vi "Wago Input Image.vi"(8 "Error In":errorcluster, 10 "Wago Data Input":T1 {"Input Process Image"."Software Constants"."Room PID Settings"."Room Dehumid Temperature I (*RM Dehum I1)" max=30000 step=1; "Input Process Image"."Software Constants"."Room PID Settings"."Room Dehumid Temperature P (*RM Dehum P1)" max=30000 step=1; "Input Process Image"."Software Constants"."Room PID Settings"."Room Cool Temperature I (*RM Cool I1)" max=30000 step=1; "Input Process Image"."Software Constants"."Room PID Settings"."Room Cool Temperature P (*RM Cool P1)" max=30000 step=1; "Input Process Image"."Software Constants"."Room PID Settings"."Room Heat I (*RM Heat I1)" max=30000 step=1; "Input Process Image"."Software Constants"."Room PID Settings"."Room Heat P (*RM Heat P1)" max=30000 step=1; "Input Process Image"."Software Constants"."Room PID Settings"."Room Humidity I (*RM Hum I1)" max=30000 step=1; "Input Process Image"."Software Constants"."Room PID Settings"."Room Humidity P (*RM Hum P1)" max=30000 step=1; "Input Process Image"."Software Constants"."Room PID Settings"."Room Dry I (*RM Dry I1)" max=30000 step=1; "Input Process Image"."Software Constants"."Room PID Settings"."Room Dry P(*RM Dry P1)" max=30000 step=1}, 11 "Modbus Master in":refnum<class "Modbus Master.lvclass">) -> (0 "Error Out":errorcluster, 2 "Wago Data Output":T1 {"Input Process Image"."Software Constants"."Room PID Settings"."Room Dehumid Temperature I (*RM Dehum I1)" max=30000 step=1; "Input Process Image"."Software Constants"."Room PID Settings"."Room Dehumid Temperature P (*RM Dehum P1)" max=30000 step=1; "Input Process Image"."Software Constants"."Room PID Settings"."Room Cool Temperature I (*RM Cool I1)" max=30000 step=1; "Input Process Image"."Software Constants"."Room PID Settings"."Room Cool Temperature P (*RM Cool P1)" max=30000 step=1; "Input Process Image"."Software Constants"."Room PID Settings"."Room Heat I (*RM Heat I1)" max=30000 step=1; "Input Process Image"."Software Constants"."Room PID Settings"."Room Heat P (*RM Heat P1)" max=30000 step=1; "Input Process Image"."Software Constants"."Room PID Settings"."Room Humidity I (*RM Hum I1)" max=30000 step=1; "Input Process Image"."Software Constants"."Room PID Settings"."Room Humidity P (*RM Hum P1)" max=30000 step=1; "Input Process Image"."Software Constants"."Room PID Settings"."Room Dry I (*RM Dry I1)" max=30000 step=1; "Input Process Image"."Software Constants"."Room PID Settings"."Room Dry P(*RM Dry P1)" max=30000 step=1}, 3 "Modbus master out":refnum<class "Modbus Master.lvclass">)   [LabVIEW 2016]
uses:
  <vilib>/NI/Modbus Library/API/Master/Modbus Master.lvclass
  Type Definitions/Wago Main Control.ctl
  Type Definitions/Wago Output Data Process Image.ctl
  Type Definitions/Wago Room Condtions.ctl
  Type Definitions/Wago Door Relays.ctl
  Type Definitions/Wago Contactor Settings.ctl
  Type Definitions/Wago Ground Leakage.ctl
  Type Definitions/Wago Input Process Image.ctl
  Type Definitions/Wago Room PID Settings.ctl
  Type Definitions/Wago Measured Input Data.ctl
  Type Definitions/Wago Room Setpoint Targets.ctl
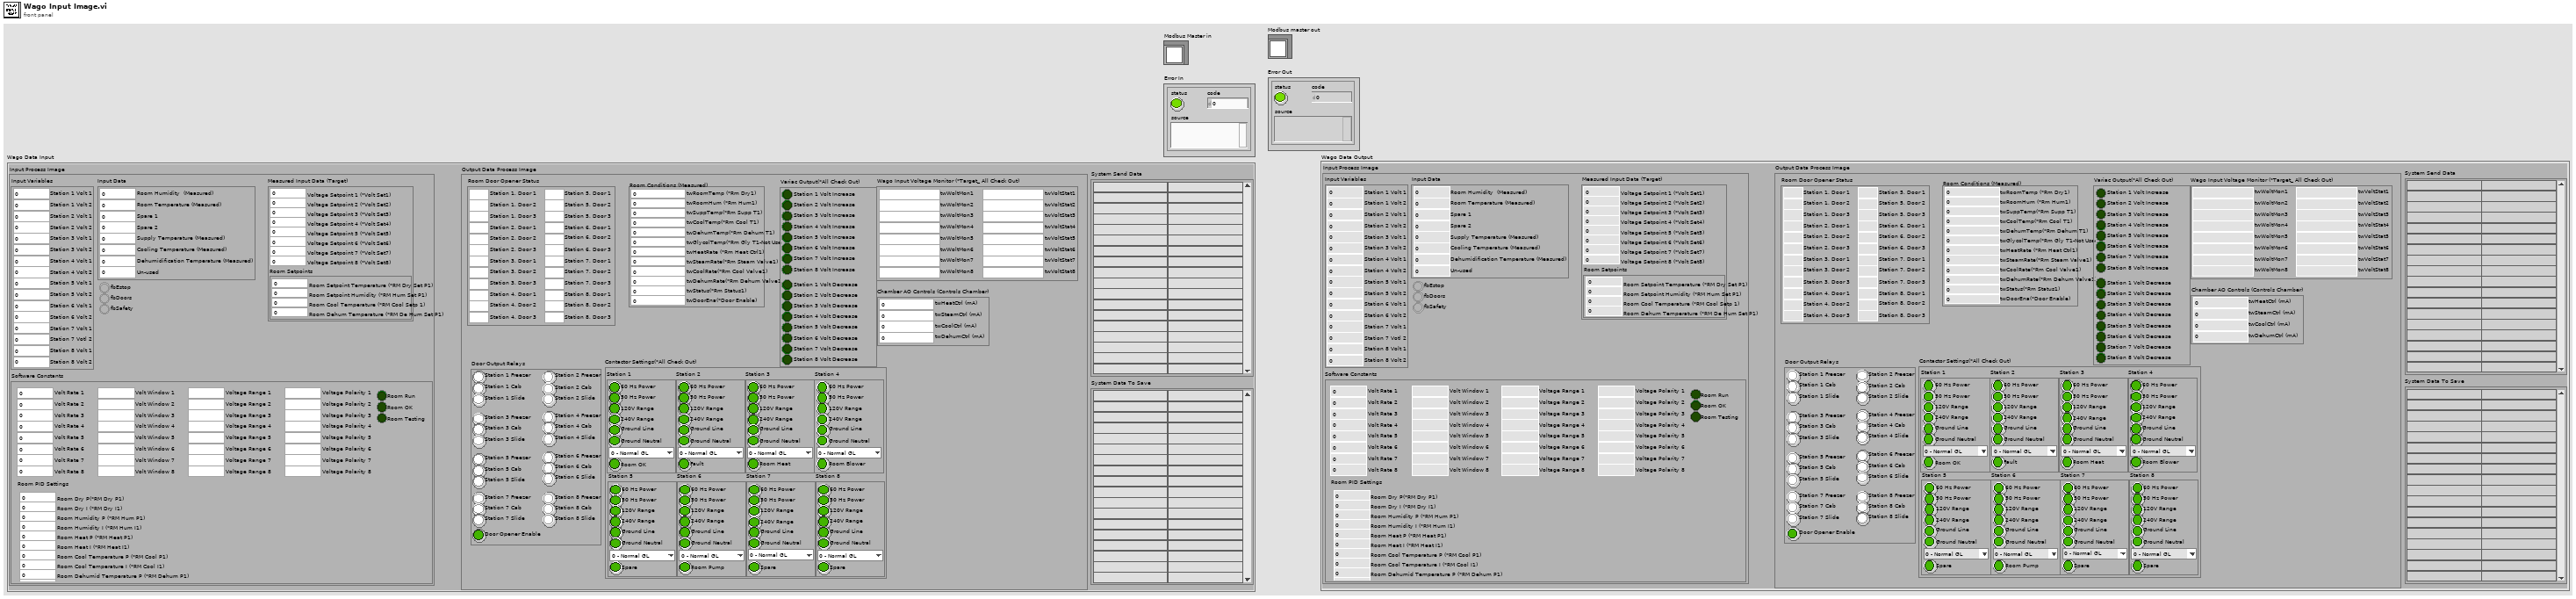
[diagram p1: front panel]
types:
  T1 = typedef "Wago Main Control.ctl" = cluster{"Output Data Process Image":T2, "Input Process Image":T7, "System Send Data":string[][], "System Data To Save":string[][]}
  T2 = typedef "Wago Output Data Process Image.ctl" = cluster{"Room Door Opener Status":cluster{"Station 1, Door 1":u16, "Station 1, Door 2":u16, "Station 1, Door 3":u16, "Station 2, Door 1":u16, "Station 2, Door 2":u16, "Station 2, Door 3":u16, "Station 3, Door 1":u16, "Station 3, Door 2":u16, "Station 3, Door 3":u16, "Station 4, Door 1":u16, "Station 4, Door 2":u16, "Station 4, Door 3":u16, "Station 5, Door 1":u16, "Station 5, Door 2":u16, "Station 5, Door 3":u16, "Station 6, Door 1":u16, "Station 6, Door 2":u16, "Station 6, Door 3":u16, "Station 7, Door 1":u16, "Station 7, Door 2":u16, "Station 7, Door 3":u16, "Station 8, Door 1":u16, "Station 8, Door 2":u16, "Station 8, Door 3":u16}, "Room Conditions (Measured)":T3, "Chamber AO Controls (Controls Chamber)":cluster{"twDehumCtrl (mA)":u16, "twCoolCtrl (mA)":u16, "twSteamCtrl (mA)":u16, "twHeatCtrl (mA)":u16}, "Variac Output(*All Check Out)":cluster{"Station 1 Volt Increase":bool, "Station 1 Volt Decrease":bool, "Station 2 Volt Increase":bool, "Station 2 Volt Decrease":bool, "Station 3 Volt Increase":bool, "Station 3 Volt Decrease":bool, "Station 4 Volt Increase":bool, "Station 4 Volt Decrease":bool, "Station 5 Volt Increase":bool, "Station 5 Volt Decrease":bool, "Station 6 Volt Increase":bool, "Station 6 Volt Decrease":bool, "Station 7 Volt Increase":bool, "Station 7 Volt Decrease":bool, "Station 8 Volt Increase":bool, "Station 8 Volt Decrease":bool}, "Door Output Relays":T4, "Wago Input Voltage Monitor (*Target_ All Check Out)":cluster{"twWoltMon1":dbl, "twWoltMon2":dbl, "twWoltMon3":dbl, "twWoltMon4":dbl, "twWoltMon5":dbl, "twWoltMon6":dbl, "twWoltMon7":dbl, "twWoltMon8":dbl, "twVoltStat1":u16, "twVoltStat2":u16, "twVoltStat3":u16, "twVoltStat4":u16, "twVoltStat5":u16, "twVoltStat6":u16, "twVoltStat7":u16, "twVoltStat8":u16}, "Contactor Settings(*All Check Out)":T5}
  T3 = typedef "Wago Room Condtions.ctl" = cluster{"twDoorEna(*Door Enable)":u16, "twStatus(*Rm Status1)":u16, "twRoomTemp (*Rm Dry1)":dbl, "twRoomHum (*Rm Hum1)":dbl, "twSuppTemp(*Rm Supp T1)":dbl, "twCoolTemp(*Rm Cool T1)":dbl, "twDehumTemp(*Rm Dehum T1)":dbl, "twGlycolTemp(*Rm Gly T1-Not Used)":dbl, "twDehumRate(*Rm Dehum Valve1)":dbl, "twCoolRate(*Rm Cool Valve1)":dbl, "twSteamRate(*Rm Steam Valve1)":dbl, "twHeatRate (*Rm Heat Ctrl1)":dbl}
  T4 = typedef "Wago Door Relays.ctl" = cluster{"Station 1 Freezer":bool, "Station 1 Cab":bool, "Station 1 Slide":bool, "Station 2 Freezer":bool, "Station 2 Cab":bool, "Station 2 Slide":bool, "Station 3 Freezer":bool, "Station 3 Cab":bool, "Station 3 Slide":bool, "Station 4 Freezer":bool, "Station 4 Cab":bool, "Station 4 Slide":bool, "Station 5 Freezer":bool, "Station 5 Cab":bool, "Station 5 Slide":bool, "Station 6 Freezer":bool, "Station 6 Cab":bool, "Station 6 Slide":bool, "Station 7 Freezer":bool, "Station 7 Cab":bool, "Station 7 Slide":bool, "Station 8 Freezer":bool, "Station 8 Cab":bool, "Station 8 Slide":bool, "Door Opener Enable":bool}
  T5 = typedef "Wago Contactor Settings.ctl" = cluster{"Station 1":cluster{"60 Hz Power":bool, "50 Hz Power":bool, "120V Range":bool, "240V Range":bool, "Ground Line":bool, "Ground Neutral":bool, "Room OK":bool, "Ground Leakage":T6}, "Station 2":cluster{"60 Hz Power":bool, "50 Hz Power":bool, "120V Range":bool, "240V Range":bool, "Ground Line":bool, "Ground Neutral":bool, "Fault":bool, "Ground Leakage":T6}, "Station 3":cluster{"60 Hz Power":bool, "50 Hz Power":bool, "120V Range":bool, "240V Range":bool, "Ground Line":bool, "Ground Neutral":bool, "Room Heat":bool, "Ground Leakage":T6}, "Station 4":cluster{"60 Hz Power":bool, "50 Hz Power":bool, "120V Range":bool, "240V Range":bool, "Ground Line":bool, "Ground Neutral":bool, "Room Blower":bool, "Ground Leakage":T6}, "Station 5":cluster{"60 Hz Power":bool, "50 Hz Power":bool, "120V Range":bool, "240V Range":bool, "Ground Line":bool, "Ground Neutral":bool, "Spare":bool, "Ground Leakage":T6}, "Station 6":cluster{"60 Hz Power":bool, "50 Hz Power":bool, "120V Range":bool, "240V Range":bool, "Ground Line":bool, "Ground Neutral":bool, "Room Pump":bool, "Ground Leakage":T6}, "Station 7":cluster{"60 Hz Power":bool, "50 Hz Power":bool, "120V Range":bool, "240V Range":bool, "Ground Line":bool, "Ground Neutral":bool, "Spare":bool, "Ground Leakage":T6}, "Station 8":cluster{"60 Hz Power":bool, "50 Hz Power":bool, "120V Range":bool, "240V Range":bool, "Ground Line":bool, "Ground Neutral":bool, "Spare":bool, "Ground Leakage":T6}}
  T6 = typedef "Wago Ground Leakage.ctl" = enum16{"0 - Normal GL", "1 - Measure GL"}
  T7 = typedef "Wago Input Process Image.ctl" = cluster{"fbEstop":bool, "fbDoors":bool, "fbSafety":bool, "Input Variables":cluster{"Station 1 Volt 1":dbl, "Station 1 Volt 2":dbl, "Station 2 Volt 1":dbl, "Station 2 Volt 2":dbl, "Station 3 Volt 1":dbl, "Station 3 Volt 2":dbl, "Station 4 Volt 1":dbl, "Station 4 Volt 2":dbl, "Station 5 Volt 1":dbl, "Station 5 Volt 2":dbl, "Station 6 Volt 1":dbl, "Station 6 Volt 2":dbl, "Station 7 Volt 1":dbl, "Station 7 Votl 2":dbl, "Station 8 Volt 1":dbl, "Station 8 Volt 2":dbl}, "Input Data":cluster{"Room Humidity  (Measured)":dbl, "Room Temperature (Measured)":dbl, "Spare 1":dbl, "Spare 2":dbl, "Supply Temperature (Measured)":dbl, "Cooling Temperature (Measured)":dbl, "Dehumidification Temperature (Measured)":dbl, "Un-used":dbl}, "Software Constants":cluster{"Volt Rate 1":u16, "Volt Rate 2":u16, "Volt Rate 3":u16, "Volt Rate 4":u16, "Volt Rate 5":u16, "Volt Rate 6":u16, "Volt Rate 7":u16, "Volt Rate 8":u16, "Volt Window 1":u16, "Volt Window 2":u16, "Volt Window 3":u16, "Volt Window 4":u16, "Volt Window 5":u16, "Volt Window 6":u16, "Volt Window 7":u16, "Volt Window 8":u16, "Voltage Range 1":u16, "Voltage Range 2":u16, "Voltage Range 3":u16, "Voltage Range 4":u16, "Voltage Range 5":u16, "Voltage Range 6":u16, "Voltage Range 7":u16, "Voltage Range 8":u16, "Voltage Polarity 1":u16, "Voltage Polarity 2":u16, "Voltage Polarity 3":u16, "Voltage Polarity 4":u16, "Voltage Polarity 5":u16, "Voltage Polarity 6":u16, "Voltage Polarity 7":u16, "Voltage Polarity 8":u16, "Room Run":bool, "Room OK":bool, "Room Testing":bool, "Room PID Settings":T8}, "Measured Input Data (Target)":T9}
  T8 = typedef "Wago Room PID Settings.ctl" = cluster{"Room Dry P(*RM Dry P1)":u16, "Room Dry I (*RM Dry I1)":u16, "Room Humidity P (*RM Hum P1)":u16, "Room Humidity I (*RM Hum I1)":u16, "Room Heat P (*RM Heat P1)":u16, "Room Heat I (*RM Heat I1)":u16, "Room Cool Temperature P (*RM Cool P1)":u16, "Room Cool Temperature I (*RM Cool I1)":u16, "Room Dehumid Temperature P (*RM Dehum P1)":u16, "Room Dehumid Temperature I (*RM Dehum I1)":u16}
  T9 = typedef "Wago Measured Input Data.ctl" = cluster{"Voltage Setpoint 1 (*Volt Set1)":dbl, "Voltage Setpoint 2 (*Volt Set2)":dbl, "Voltage Setpoint 3 (*Volt Set3)":dbl, "Voltage Setpoint 4 (*Volt Set4)":dbl, "Voltage Setpoint 5 (*Volt Set5)":dbl, "Voltage Setpoint 6 (*Volt Set6)":dbl, "Voltage Setpoint 7 (*Volt Set7)":dbl, "Voltage Setpoint 8 (*Volt Set8)":dbl, "Room Setpoints":T10}
  T10 = typedef "Wago Room Setpoint Targets.ctl" = cluster{"Room Setpoint Temperature (*RM Dry Set P1)":dbl, "Room Setpoint Humidity (*RM Hum Set P1)":dbl, "Room Cool Temperature (*RM Cool Setp 1)":dbl, "Room Dehum Temperature (*RM De Hum Set P1)":dbl}
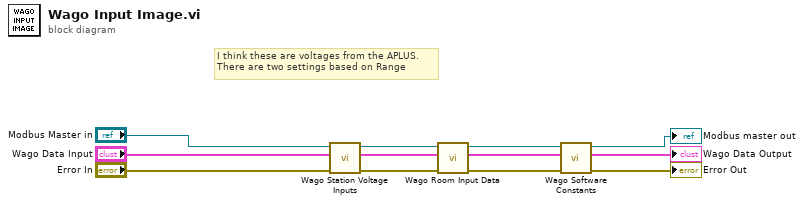
[diagram p0: block diagram]
diagram:
  # "I think these are voltages from the APLUS.\nThere are two settings based on Range"
  n1 = call "Wago Station Voltage Inputs.vi"("error in (no error)"="Error In", "Wago Data Input"="Wago Data Input", "Modbus Master in"="Modbus Master in") -> ("error out"=w9:errorcluster, "Wago Data Output"=w8:T1, "Modbus Master out"=w7:refnum<class "Modbus Master.lvclass">)  [unwired: 6 in]
  n2 = call "Wago Room Input Data.vi"("Error In"=w9, "Wago Data Input"=w8, "Modbus Master in"=w7) -> ("error out"=w6:errorcluster, "Wago Data Output"=w4:T1, "Modbus Master out"=w2:refnum<class "Modbus Master.lvclass">)  [unwired: 6 in]
  n3 = call "Wago Software Constants.vi"("Error In"=w6, "Wago Data Input"=w4, "Modbus Master in"=w2) -> ("Error Out"=→"Error Out":errorcluster, "Wago Data Output"=→"Wago Data Output":T1, "Modbus Master out"=→"Modbus master out":refnum<class "Modbus Master.lvclass">)  [unwired: 6 in]
